vi "Connect OPC UA.vi"(6 "Trial Number":i32=3, 7 "timeout(s)":T3=5, 8 "error in":errorcluster, 9 "Sequence Context":refnum<k7>, 10 "URL":string="opc.tcp://DESKTOP-T6QR0HI:4991/LunarTester", 11 "OPC UA In":refnum<class "OPC UA.lvclass">) -> (0 "error out":errorcluster={"status"=TRUE, "code"=97, "source"="Unknown System Error in TestStand - Initialize Termination Monitor.vi->Login Progress.vi"}, 2 "OPC UA refnum":T1, 3 "OPC UA out":refnum<class "OPC UA.lvclass">)   [LabVIEW 2019, in "OPC UA.lvlib" / "OPC UA.lvclass"]
uses:
  OPC UA.lvclass
  <vilib>/OPCUA/controls/Time Out.ctl
  OPC UA.lvclass/OPC UA.ctl
  <vilib>/OPCUA/NI OPC UA Client.lvlib
  <vilib>/OPCUA/controls/OPC UA Client Refnum.ctl
panel:
  out "Waiting Lights":T2
  out "Trial":i32
  out "stop":bool
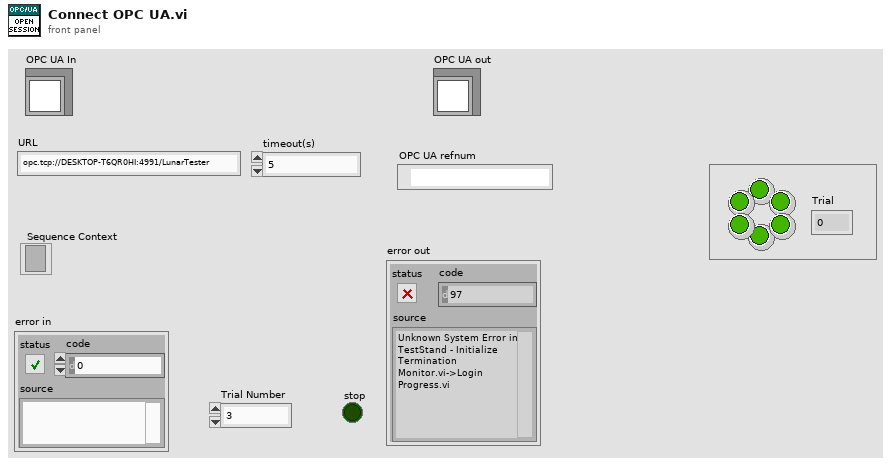
[diagram p1: front panel]
types:
  T1 = typedef "OPC UA Client Refnum.ctl" = refnum<k21>
  T2 = cluster{"wait 1":bool, "wait 2":bool, "wait 3":bool, "wait 4":bool, "wait 5":bool, "wait 6":bool}
  T3 = typedef "Time Out.ctl" = u32
  T4 = typedef "TestStand - Status Monitor.ctl" = cluster{"Sequence Context":refnum<k7>, "Execution":refnum<k7>, "Termination Monitor":refnum<k7>}
  T5 = cluster{"[0]":bool, "[1]":bool, "[2]":bool, "[3]":bool, "[4]":bool, "[5]":bool}
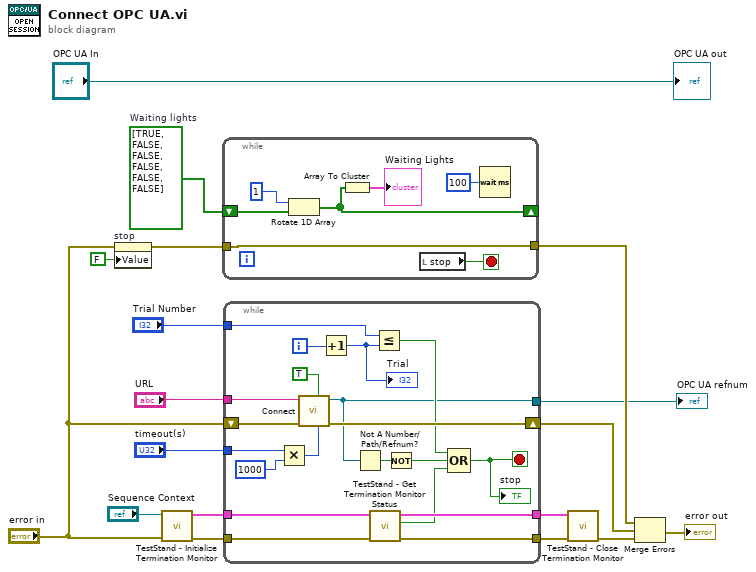
[diagram p0: block diagram]
diagram:
  w9 = bool[] [TRUE, FALSE, FALSE, FALSE, FALSE, FALSE]  # Waiting lights
  n1 = property on="stop" class="Bool (strict)"(error in="error in", "Value"=FALSE ("stop")) -> (error out=w8:errorcluster)  [unwired: 1 in, 1 out]
  n2 = call <vilib>:"TestStand - Initialize Termination Monitor.vi"("error in (no error)"="error in", "Sequence Context In"="Sequence Context") -> ("error out"=w13:errorcluster, "Status Monitor Out"=w14:T4)  [unwired: 8 in]
  n3 = while {
    tunnel: w8 -> [w23]
    tunnel: [w23] -> w7
    shift-right: [w20] -> _
    shift-left: w9 -> [w21]
    stop <- w24 stop-if-true
    n4 = Rotate 1D Array(1:w21, 2:1 ("n")) -> (0:w20:bool[])
    n5 = Array To Cluster(array=w20) -> (cluster=→"Waiting Lights":T5)
    n6 = local read "stop"() -> (w24:bool)
    n7 = Wait (ms)(milliseconds to wait=u32 100) -> ()  [unwired: 1 out]
  }
  n8 = while {
    tunnel: "URL" -> [w43]
    tunnel: w13 -> [w41]
    tunnel: w14 -> [w42]
    tunnel: [w40] -> w15
    tunnel: [w39] -> w16
    tunnel: "timeout(s)" -> [w38]
    shift-right: [w33] -> w5
    shift-left: "error in" -> [w44]
    tunnel: "Trial Number" -> [w28]
    tunnel: [w26] -> w1
    i -> [w35]
    stop <- w29 stop-if-true
    n9 = Multiply(x=w38, y=T3 1000) -> (x*y=w37:T3)
    n10 = call <vilib>:"Connect.vi"("timeout (5000 ms)"=w37, "trust any server (F)"=TRUE, "error in (no error)"=w44, "server endpoint URL"=w43) -> ("error out"=w33:errorcluster, "OPC UA client refnum out"=w26:T1)  [unwired: 5 in, 1 out]
    n11 = Increment(x=w35) -> (x+1=w34:i32)
    "Trial" <- w34
    n12 = Not A Number/Path/Refnum?(number/path/refnum=w26) -> (NaN/Path/Refnum?=w32:bool)
    n13 = call <vilib>:"TestStand - Get Termination Monitor Status.vi"("error in (no error)"=w41, "Status Monitor In"=w42) -> ("error out"=w39:errorcluster, "Terminating or Aborting"=w30:bool, "Status Monitor Out"=w40:T4)  [unwired: 7 in]
    n14 = Less Or Equal?(x=w28, y=w34) -> (x <= y?=w31:bool)
    n15 = Not(x=w32) -> (.not. x?=w27:bool)
    n16 = Compound Arithmetic op=OR(w31, w27, w30) -> (w29:bool)
    "stop" <- w29
  }
  "OPC UA refnum" <- w1
  n17 = call <vilib>:"TestStand - Close Termination Monitor.vi"("error in (no error)"=w16, "Status Monitor In"=w15) -> ("error out"=w17:errorcluster)  [unwired: 9 in]
  n18 = Merge Errors(w7, w5, w17) -> (→"error out":errorcluster)
  "OPC UA out" <- "OPC UA In"
